vi "Build_Read Input Registers.vi"(8 "error in (no error)":errorcluster, 9 "quantity":u16, 10 "starting address":u16) -> (0 "error out":errorcluster, 3 "MB_PDU":T1={"Function Code"=1, "Data"=[], "RTU_DataBytes"=0})   [LabVIEW 2012, in "MB Master.lvlib"]
doc: "Builds PDU for Read Input Registers (function code 4)."
uses:
  MB Master.lvlib
  MB_PDU_Cluster.ctl
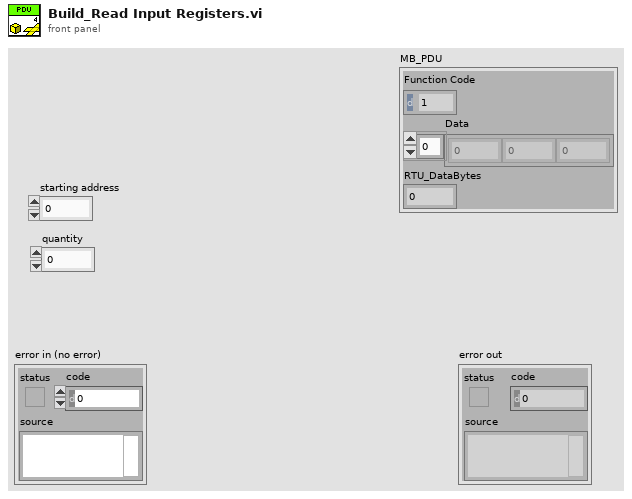
[diagram p1: front panel]
types:
  T1 = typedef "MB Master.lvlib/MB_PDU_Cluster.ctl" = cluster{"Function Code":u8, "Data":u8[], "RTU_DataBytes":i32}
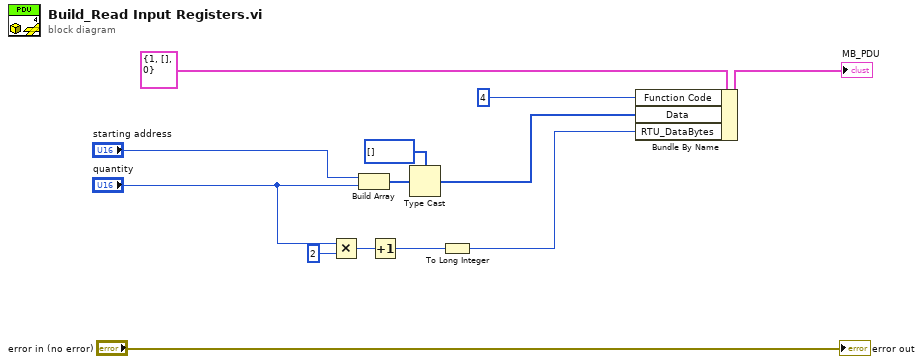
[diagram p0: block diagram]
diagram:
  n1 = Multiply(x="quantity", y=u16 2) -> (x*y=w4:u16)
  n2 = Build Array("starting address", "quantity") -> (w13:u16[])
  n3 = Increment(x=w4) -> (x+1=w3:u16)
  n4 = Type Cast(type=u8[] [], x=w13) -> (*(type *) &x=w8:u8[])
  n5 = To Long Integer(number=w3) -> (32bit integer=w1:i32)
  n6 = Bundle By Name(cluster=T1 {"Function Code"=1, "Data"=[], "RTU_DataBytes"=0} ("Modbus Serial New.lvlib:MB_PDU.lvclass"), "Function Code"=u8 4, "Data"=w8, "RTU_DataBytes"=w1) -> (→"MB_PDU":T1)
  "error out" <- "error in (no error)"
